vi "Authorization_response.vi"() -> ()   [LabVIEW 2016]
panel:
  out "headers 2":string="HTTP/1.1 401 Unauthorized\r\nWWW-Authenticate: Digest realm=\"Login to 4H0572FPAG801C6\", qop=\"auth\", nonce=\"1006650171\", opaque=\"a663b9f7478c0416c2eaa1c598bca2154a0b27af\"\r\nConnection: close\r\nCONTENT-LENGTH: 0\r\n\r\nHTTP/1.1 401 Unauthorized\r\nConnection: close\r\nContent-type: text/plain;charset=utf-8\r\nContent-Length: 27\r\n\r\n"
  out "headers":string="HTTP/1.1 401 Unauthorized\r\nWWW-Authenticate: Digest realm=\"Login to 4H0572FPAG801C6\", qop=\"auth\", nonce=\"341160736\", opaque=\"a663b9f7478c0416c2eaa1c598bca2154a0b27af\"\r\nConnection: close\r\nCONTENT-LENGTH: 0\r\n\r\nHTTP/1.1 200 OK\r\nContent-type: text/plain;charset=utf-8\r\nCONNECTION: close\r\nCONTENT-LENGTH: 9469\r\n\r\n"
  # "LV Send_CGI_Strings.vi con password corretta"
  # "LV Send_CGI_Strings.vi con password sbagliata"
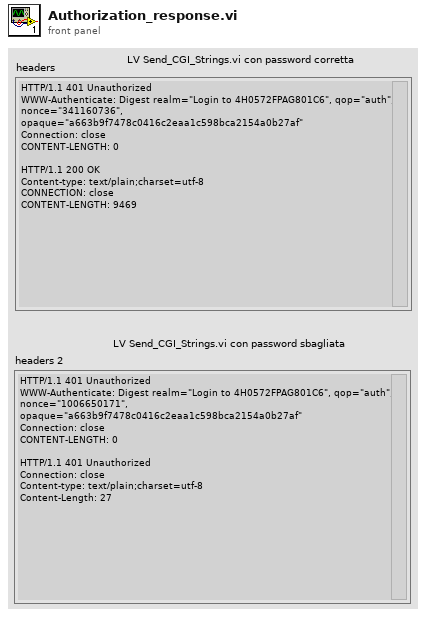
[diagram p1: front panel]
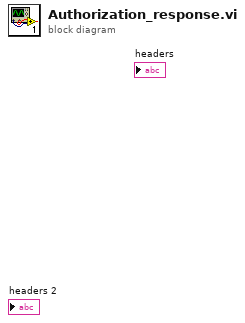
[diagram p0: block diagram]
diagram:
